vi "LOG_Initialize.vi"(8 "error in (no error)":errorcluster, 11 "max queue size (500)":i32=500) -> (0 "error out":errorcluster, 3 "Message queue out":refnum<queue>)   [LabVIEW 2015]
uses:
  Controls/LOG_MessageQueue.ctl
  Controls/GFV Action.ctl
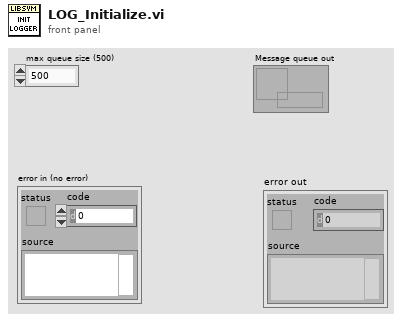
[diagram p1: front panel]
types:
  T1 = typedef "GFV Action.ctl" = enum16{"Get", "Set", "Delete"}
  T2 = typedef "LOG_MessageQueue.ctl" = cluster{"Time":timestamp, "message":string}
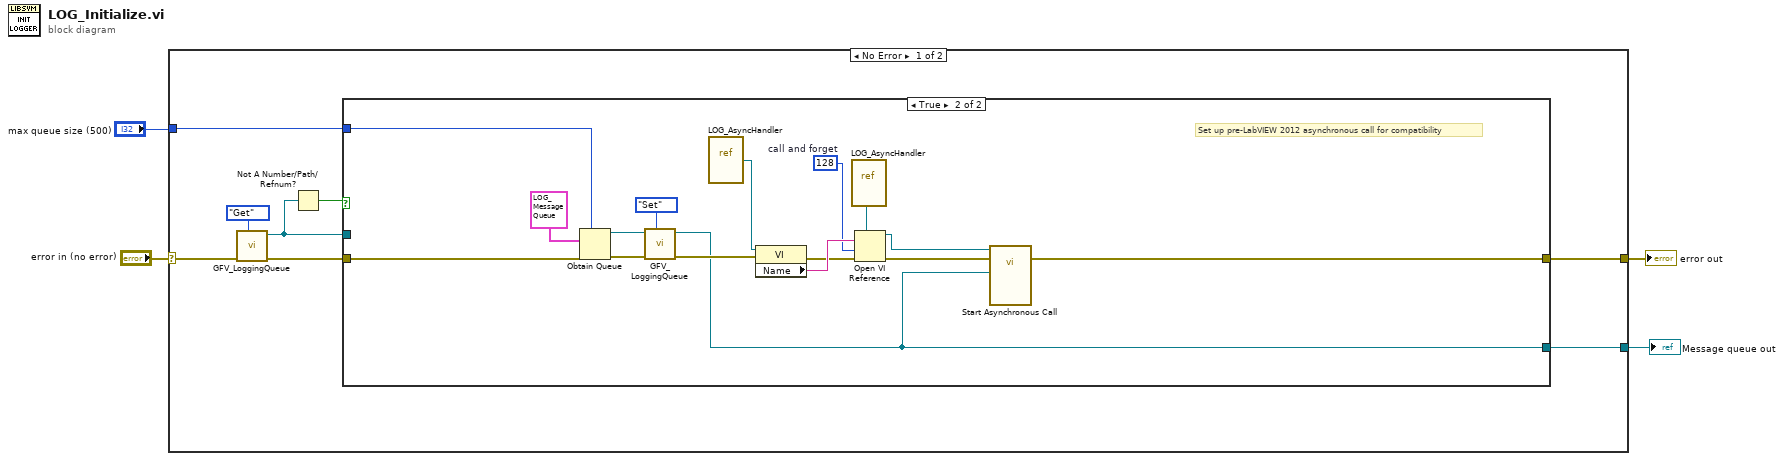
[diagram p0: block diagram]
diagram:
  n1 = case shown="No Error" "error in (no error)" {
    selector: "error in (no error)" -> [w9 w31]
    tunnel: "max queue size (500)" -> [w10 _]
    tunnel: [w12 w31] -> w2
    tunnel: [w11 _] -> w1
    frame No Error {
      n2 = call "GFV_LoggingQueue.vi"("GFV Action"=GFV_Action."Get", "error in (no error)"=w9) -> ("error out"=w8:errorcluster, "Message queue out"=w5:refnum<queue>)  [unwired: 8 in]
      n3 = Not A Number/Path/Refnum?(number/path/refnum=w5) -> (NaN/Path/Refnum?=w7:bool)
      n4 = case shown="True" w7 {
        tunnel: [w14 w15] -> w12
        tunnel: w8 -> [w14 w21]
        tunnel: [w13 w16] -> w11
        tunnel: w10 -> [_ w22]
        tunnel: w5 -> [w13 _]
        frame False {
        }
        frame True {
          w29 = 128  # call and forget
          # "Set up pre-LabVIEW 2012 asynchronous call for compatibility"
          n5 = Obtain Queue(max queue size (-1, unlimited)=w22, element data type=T2 {"Time"=timestamp(0 s since 1904-01-01), "message"=""} ("Log Event"), error in (no error)=w21) -> (queue out=w27:refnum<queue>, error out=w25:errorcluster)  [unwired: 2 in, 1 out]
          n6 = call "GFV_LoggingQueue.vi"("GFV Action"=GFV_Action."Set", "error in (no error)"=w25, "Message queue in"=w27) -> ("error out"=w23:errorcluster, "Message queue out"=w16:refnum<queue>)  [unwired: 7 in]
          n7 = vi-ref "LOG_AsyncHandler.vi"() -> (w20:refnum<vi>)
          n8 = property class="VI"(reference=w20, error in=w23) -> (error out=w28:errorcluster, "Name"=w30:string)  [unwired: 1 out]
          n9 = vi-ref "LOG_AsyncHandler.vi"() -> (w19:refnum<vi>)
          n10 = Open VI Reference(type specifier VI Refnum (for type only)=w19, vi path=w30, options=w29, error in (no error)=w28) -> (vi reference=w17:refnum<vi>, error out=w18:errorcluster)  [unwired: 2 in]
          n11 = call-by-ref "Start Asynchronous Call"(reference=w17, error in=w18, "Message queue in"=w16) -> (error out=w15:errorcluster)  [unwired: 10 in, 2 out]
        }
      }
    }
    frame Error {
    }
  }
  "error out" <- w2
  "Message queue out" <- w1
